vi "Intensity Graph to Igor Graph.vi"(8 "error in (no error)":errorcluster, 9 "Notes":string, 10 "Intensity Graph Reference":refnum<vi>, 11 "Path":path=path "C:/temp") -> (0 "error out":errorcluster, 3 "file":path)   [LabVIEW 2019, in "LV-Data.ITX.lvclass"]
uses:
  LV-Data.ITX.lvclass
  <userlib>/LevyLab/Graph Utilities/graph_utilities.lvclass/graph_utilities.ctl
  <userlib>/LevyLab/Graph Utilities/graph_utilities.lvclass
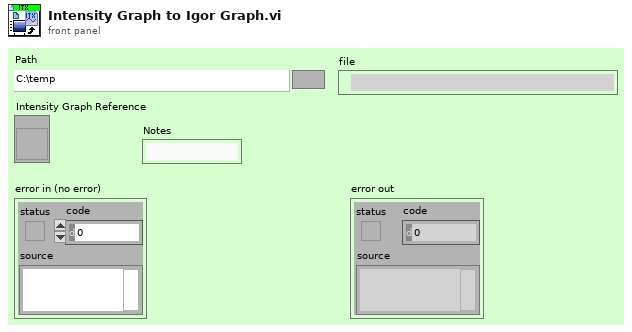
[diagram p1: front panel]
types:
  T1 = cluster{"Value":dbl[][], "X Scale":dbl[], "Y Scale":dbl[]}
  T2 = cluster{"ZScale.Minimum":dbl, "ZScale.Maximum":dbl}
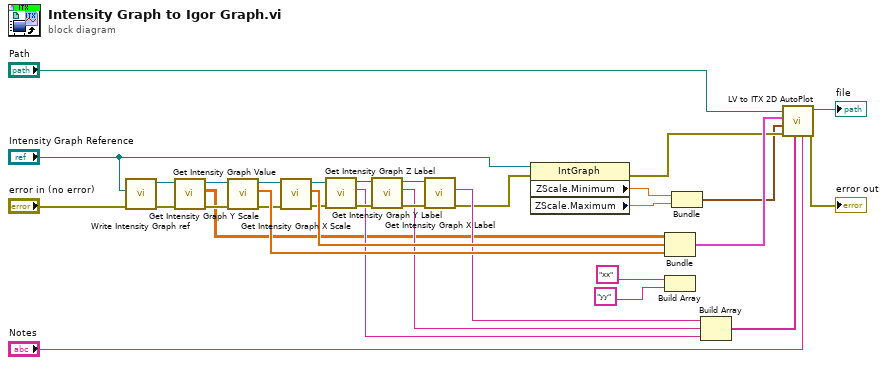
[diagram p0: block diagram]
diagram:
  n1 = call <userlib>:"Write Intensity Graph ref.vi"("error in (no error)"="error in (no error)", "Intensity Graph"="Intensity Graph Reference") -> ("error out"=w30:errorcluster, "graph_utilities out"=w31:refnum<class "graph_utilities.lvclass">)  [unwired: 8 in]
  n2 = call <userlib>:"Get Intensity Graph Value.vi"("error in (no error)"=w30, "graph_utilities in"=w31) -> ("error out"=w27:errorcluster, "Value"=w13:dbl[][], "graph_utilities out"=w28:refnum<class "graph_utilities.lvclass">)  [unwired: 7 in]
  n3 = call <userlib>:"Get Intensity Graph Y Scale.vi"("error in (no error)"=w27, "graph_utilities in"=w28) -> ("error out"=w24:errorcluster, "Y Scale"=w26:dbl[], "graph_utilities out"=w25:refnum<class "graph_utilities.lvclass">)  [unwired: 6 in, 1 out]
  n4 = call <userlib>:"Get Intensity Graph X Scale.vi"("error in (no error)"=w24, "graph_utilities in"=w25) -> ("error out"=w19:errorcluster, "X Scale"=w29:dbl[], "graph_utilities out"=w18:refnum<class "graph_utilities.lvclass">)  [unwired: 6 in, 1 out]
  n5 = call <userlib>:"Get Intensity Graph Z Label.vi"("error in (no error)"=w19, "graph_utilities in"=w18) -> ("error out"=w21:errorcluster, "Z Label"=w15:string, "graph_utilities out"=w20:refnum<class "graph_utilities.lvclass">)  [unwired: 7 in]
  n6 = call <userlib>:"Get Intensity Graph Y Label.vi"("error in (no error)"=w21, "graph_utilities in"=w20) -> ("error out"=w23:errorcluster, "Y Label"=w16:string, "graph_utilities out"=w22:refnum<class "graph_utilities.lvclass">)  [unwired: 7 in]
  n7 = call <userlib>:"Get Intensity Graph X Label.vi"("error in (no error)"=w23, "graph_utilities in"=w22) -> ("error out"=w5:errorcluster, "X Label"=w17:string)  [unwired: 7 in, 1 out]
  n8 = property on="Property Node" class="IntGraph"(reference="Intensity Graph Reference", error in=w5) -> (error out=w4:errorcluster, "ZScale.Minimum"=w3:dbl, "ZScale.Maximum"=w2:dbl)  [unwired: 1 out]
  n9 = Bundle("Value"=w13, "X Scale"=w29, "Y Scale"=w26) -> (w9:T1)  [unwired: 1 in]
  n10 = Build Array("xx" ("X Scale.Name Label.Text"), "yy" ("X Scale.Name Label.Text")) -> ()  [unwired: 1 out]
  n11 = Bundle("ZScale.Minimum"=w3, "ZScale.Maximum"=w2) -> (w1:T2)  [unwired: 1 in]
  n12 = Build Array(w17, w16, w15) -> (w12:string[])
  n13 = call "LV to ITX 2D AutoPlot.vi"("Notes"="Notes", "X,Y,Z Labels"=w12, "error in"=w4, "Z Range"=w1, "2D, X, Y (Cluster)"=w9, "path"="Path") -> ("error out"=→"error out":errorcluster, "file"=→"file":path)  [unwired: 4 in]
